vi "Update their Tulip.vi"(8 "Data file":string, 10 "Test pass?":bool=TRUE, 11 "Serial number":string) -> (0 "error out":errorcluster, 1 "Status String":string, 2 "Not Found?":bool, 3 "Response body":string)   [LabVIEW 2021]
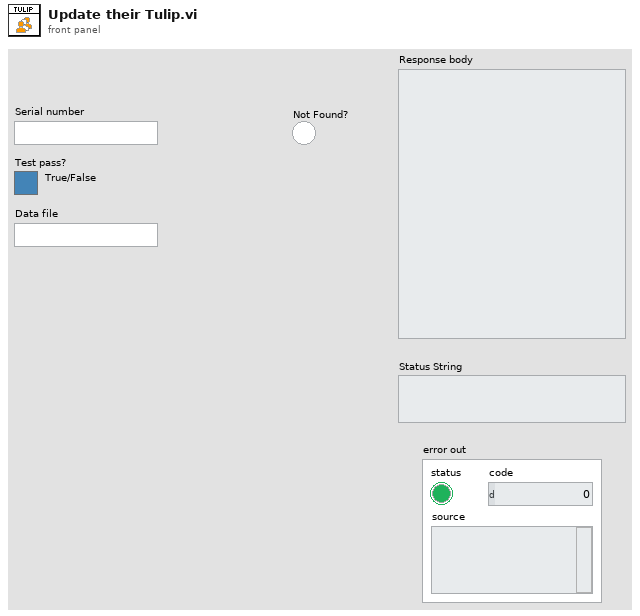
[diagram p1: front panel]
types:
  T1 = cluster{"rtppi_assembly_test_pass":bool, "revmq_functional_testing_file":string}
  T2 = enum16{"Init", "Get headers", "Get", "Post", "Put", "Close"}
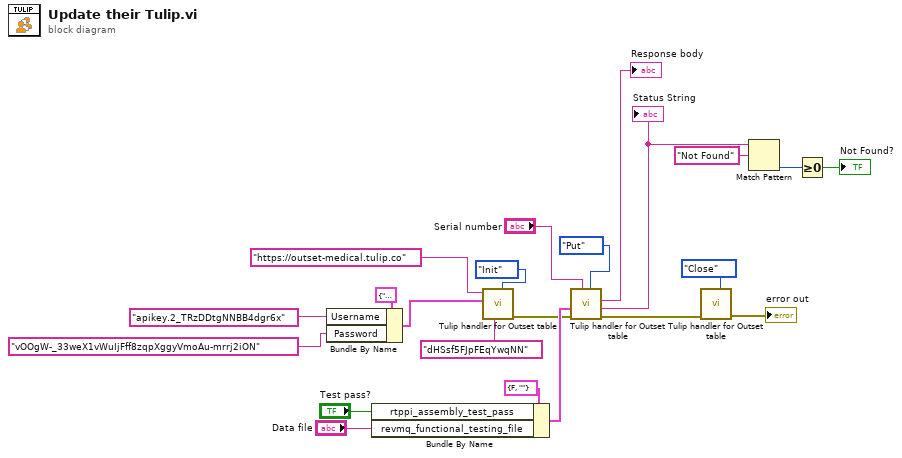
[diagram p0: block diagram]
diagram:
  n1 = Bundle By Name(cluster=cluster{"Username":string, "Password":string} {"Username"="apikey.2_WNWgDzkcRL7LwQrSC", "Password"="uUTRYqQF2kxie-OG2NdFiDN_Ok5rwnamrdCqWvd0OVz"} ("Authentication"), "Username"="apikey.2_TRzDDtgNNBB4dgr6x", "Password"="vOOgW-_33weX1vWuIjFff8zqpXggyVmoAu-mrrj2iON") -> (w20:cluster{"Username":string, "Password":string})
  n2 = Bundle By Name(cluster=T1 {"rtppi_assembly_test_pass"=FALSE, "revmq_functional_testing_file"=""} ("Body"), "rtppi_assembly_test_pass"="Test pass?", "revmq_functional_testing_file"="Data file") -> (w6:T1)
  n3 = call "Tulip handler for Outset table.vi"("State"=T2."Init", "Table ID"="dHSsf5FJpFEqYwqNN", "Authentication"=w20, "URL"="https://outset-medical.tulip.co") -> ("error out"=w5:errorcluster)  [unwired: 5 in, 2 out]
  n4 = call "Tulip handler for Outset table.vi"("State"=T2."Put", "Part ID"="Serial number", "error in"=w5, "Body"=w6) -> ("error out"=w15:errorcluster, "Status String"=w4:string, "Response body"=→"Response body":string)  [unwired: 5 in]
  "Status String" <- w4
  n5 = call "Tulip handler for Outset table.vi"("State"=T2."Close", "error in"=w15) -> ("error out"=→"error out":errorcluster)  [unwired: 7 in, 2 out]
  n6 = Match Pattern(string=w4, regular expression="Not Found") -> (offset past match=w2:i32)  [unwired: 1 in, 3 out]
  n7 = Greater Or Equal To 0?(x=w2) -> (x >= 0?=→"Not Found?":bool)
